vi "rs3 get_raw_data_size.vi"(8 "error in (no error)":errorcluster, 10 "PointToBuffer":u64) -> (0 "error out":errorcluster, 1 "error":u64, 3 "size":i32)   [LabVIEW 2017, in "libRealSense3.lvlib"]
doc: "STARTS the streaming of a specific sensor, based on the input QUEUE."
uses:
  libRealSense3.lvlib
  realsense2.dll
panel:
  # "RS get raw data size"
  # "(C) 2019 Intel Corp.,  AGJ"
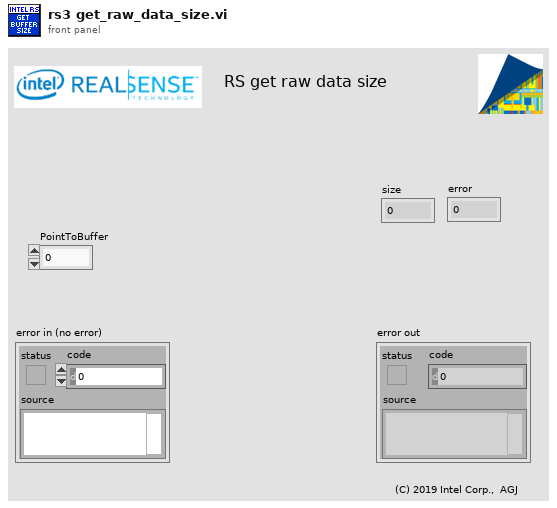
[diagram p1: front panel]
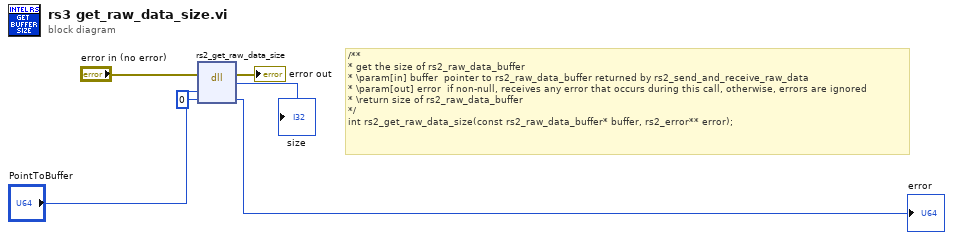
[diagram p0: block diagram]
diagram:
  # "/**\n* get the size of rs2_raw_data_buffer\n* \\param[in] buffer  pointer to rs2_raw_data_buffer returned by rs2_send_and_receive_raw_data\n* \\param[out] error  if non-null, receives any error that occurs during this call, otherwise, errors are ignored\n* \\return size of rs2_raw_data_buffer\n*/\nint rs2_get_raw_data_size(const rs2_raw_data_buffer* buffer, rs2_error** error);"
  n1 = dll-call lib="C:/Users/agrunnet/Documents/libRealSense6/realsense2.dll" fn="rs2_get_raw_data_size"(error in="error in (no error)", "PointToBuffer"="PointToBuffer", "error"=u64 0) -> (error out=→"error out":errorcluster, "size"=→"size":i32, "error"=→"error":u64)  [unwired: 3 in, 1 out]
